vi "Zero Crossing PtByPt.vi"(1 "initialize":bool, 2 "direction":enum16{"either", "minus-plus", "plus-minus"}(ring), 3 "input data point":dbl format="%0.2f") -> (0 "crossing":bool)   [LabVIEW 2017, in "NI_PtbyPt.lvlib"]
doc: "Detects zero crossings of <B>input data point</B>. <B>crossing</B> becomes TRUE immediately after the transition occurs."
uses:
  <vilib>/ptbypt/NI_PtbyPt.lvlib
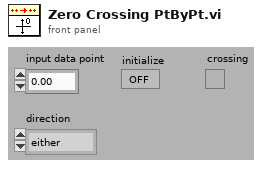
[diagram p1: front panel]
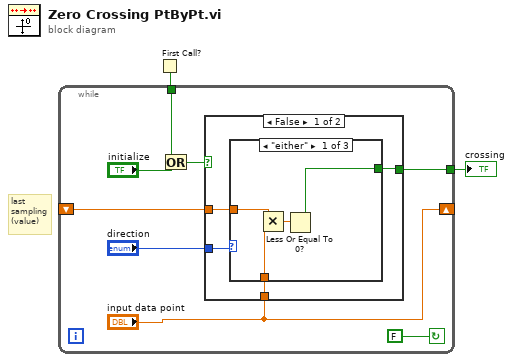
[diagram p0: block diagram]
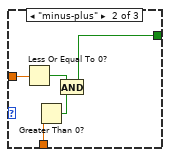
[diagram p2: hidden frame]
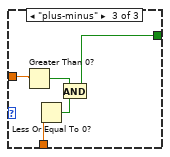
[diagram p3: hidden frame]
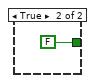
[diagram p4: hidden frame]
diagram:
  # "last\nsampling\n(value)"
  n1 = First Call?() -> (First Call?: T/F=w1:bool)
  n2 = while {
    tunnel: w1 -> [w3]
    tunnel: [w10] -> w2
    shift-left: _ -> [w8]
    shift-right: ["input data point"] -> _
    stop <- FALSE continue-if-true
    n3 = Or(x=w3, y="initialize") -> (x .or. y?=w5:bool)
    n4 = case shown="False" w5 {
      tunnel: [w11 FALSE] -> w10
      tunnel: "direction" -> [w14 _]
      tunnel: w8 -> [w13 _]
      tunnel: "input data point" -> [w12 _]
      frame False {
        n5 = case shown="\"either\"" w14 {
          tunnel: w13 -> [w18 w23 w28]
          tunnel: w12 -> [w17 w22 w24]
          tunnel: [w15 w19 w25] -> w11
          frame "either" {
            n6 = Multiply(x=w18, y=w17) -> (x*y=w16:dbl)
            n7 = Less Or Equal To 0?(x=w16) -> (x <= 0?=w15:bool)
          }
          frame "minus-plus" {
            n8 = Less Or Equal To 0?(x=w23) -> (x <= 0?=w21:bool)
            n9 = Greater Than 0?(x=w22) -> (x > 0?=w20:bool)
            n10 = And(x=w21, y=w20) -> (x .and. y?=w19:bool)
          }
          frame "plus-minus" {
            n11 = Greater Than 0?(x=w28) -> (x > 0?=w27:bool)
            n12 = Less Or Equal To 0?(x=w24) -> (x <= 0?=w26:bool)
            n13 = And(x=w27, y=w26) -> (x .and. y?=w25:bool)
          }
        }
      }
      frame True {
      }
    }
  }
  "crossing" <- w2
